vi "FTW-TestExecutive-Sequence-Interpret.vi"(0 "JSON":string, 11 "error in":errorcluster) -> (4 "Sequence":T1[](array[typedef]) {"Results"."Start Time" format="%<%Y-%m-%d %H:%M:%S%03u>T"; "Results"."Elapsed Time" format="%<%H:%M:%S%3u>t"; "Elapsed Time" format="%<%H:%M:%S%3u>t"}, 15 "error out":errorcluster)   [LabVIEW 2015]
doc: "Can be used to interpret the following messages\n\nSequenceLoaded\nSequenceComplete\nStepChange"
uses:
  FTW-TestExecutive-Step.ctl
  FTW-TestExecutive-Step-State.ctl
  FTW-TestExecutive-Results.ctl
  source/JSON/core/FTW-JSON-Core-EncodingFlags.vi
  source/JSON/FTW-JSON-Parse.vi
  source/Reflection/FTW-Reflection-Type.vi
  source/CodeGen/JSON Deserialize/FTW-JSON-Core-GetFlattenedValue.vi
  source/CodeGen/JSON Deserialize/FTW-JSON-Deserialize.xnode
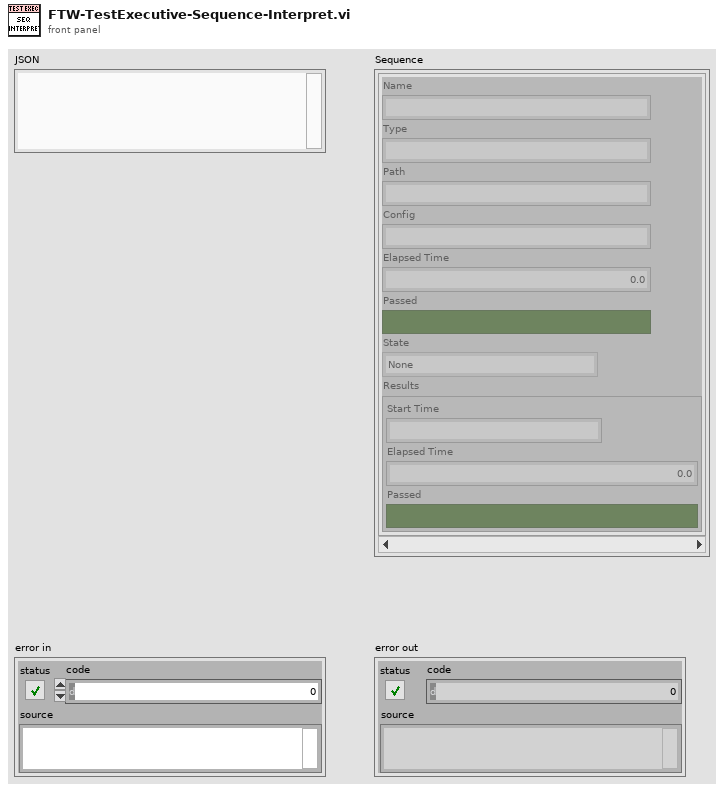
[diagram p1: front panel]
types:
  T1 = typedef "FTW-TestExecutive-Step.ctl" = cluster{"Name":string, "Type":string, "Path":string, "Config":string, "Elapsed Time":dbl, "Passed":bool, "State":T2, "Results":T3}
  T2 = typedef "FTW-TestExecutive-Step-State.ctl" = enum8{"None", "Failed", "Passed", "Timed out", "Aborted"}
  T3 = typedef "FTW-TestExecutive-Results.ctl" = cluster{"Start Time":timestamp, "Elapsed Time":dbl, "Passed":bool}
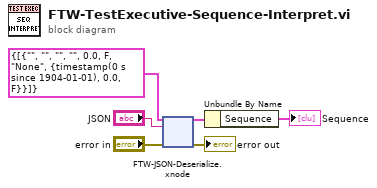
[diagram p0: block diagram]
diagram:
  n1 = xnode "FTW-JSON-Deserialize.xnode"("Type and Defaults"=cluster{"Sequence":T1[]} {"Sequence"=[{"Name"="", "Type"="", "Path"="", "Config"="", "Elapsed Time"=0.0, "Passed"=FALSE, "State"=enum."None", "Results"={"Start Time"=timestamp(0 s since 1904-01-01), "Elapsed Time"=0.0, "Passed"=FALSE}}]}, "JSON String"="JSON", "error in"="error in") -> ("Values"=w3:cluster{"Sequence":T1[]}, "error out"=→"error out":errorcluster)
  n2 = Unbundle By Name(w3) -> ("Sequence"=→"Sequence":T1[])
